vi "PH_Sound.open or close Microfone.vi"(0 "i ref in":refnum<vi>, 2 "Action":u16(ring) items=["Open", "Close"], 5 "error in (no error)":errorcluster) -> (14 "i ref out":refnum<vi>, 19 "error out":errorcluster)   [LabVIEW 2014, in "PH_Sound.lvlib"]
doc: "If the related Tagname is not N/A, this VI switches sets a Beckhoff-value to open or close the microfone."
uses:
  PH_Sound.lvlib
  PH_Devices/PH_Beckhoff/PH_Beckhoff.lvlib
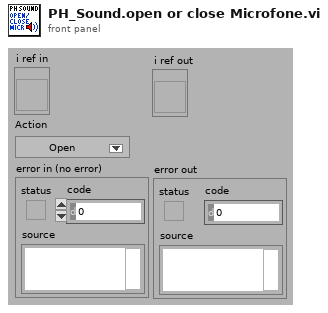
[diagram p1: front panel]
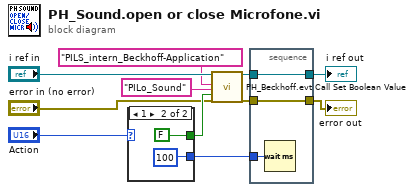
[diagram p0: block diagram]
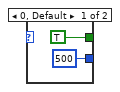
[diagram p2: hidden frame]
diagram:
  n1 = case shown="1" "Action" {
    tunnel: [TRUE FALSE] -> w7
    tunnel: [u32 500 ("milliseconds to wait") u32 100 ("milliseconds to wait")] -> w8
    frame 0, Default {
    }
    frame 1 {
    }
  }
  n2 = call "PH_Beckhoff.evt Call Set Boolean Value.vi"("i ref in"="i ref in", "Beckhoff Instance"="PILS_intern_Beckhoff-Application", "Tagname to set"="PILo_Sound" ("DIM Service Name Open Micro"), "Value"=w7, "error in"="error in (no error)") -> ("i ref out"=w5:refnum<vi>, "error out"=w6:errorcluster)  [unwired: 13 in]
  n3 = stacked-sequence {
    tunnel: w5 -> [w18]
    tunnel: [w18] -> w10
    tunnel: w6 -> [w17]
    tunnel: [w17] -> w11
    tunnel: w8 -> [w16]
    frame #0 {
      n4 = Wait (ms)(milliseconds to wait=w16) -> ()  [unwired: 1 out]
    }
  }
  "error out" <- w11
  "i ref out" <- w10
